vi "Set Temp Value.vi"(8 "error in (no error)":errorcluster, 10 "Temp.":dbl, 11 "Central Control in":refnum<class "Central Control.lvclass">) -> (0 "error out":errorcluster, 3 "Central Control out":refnum<class "Central Control.lvclass">)   [LabVIEW 2021, in "Central Control.lvlib" / "Central Control.lvclass"]
uses:
  Central Control.lvclass
  Central Control.lvclass/Central Control.ctl
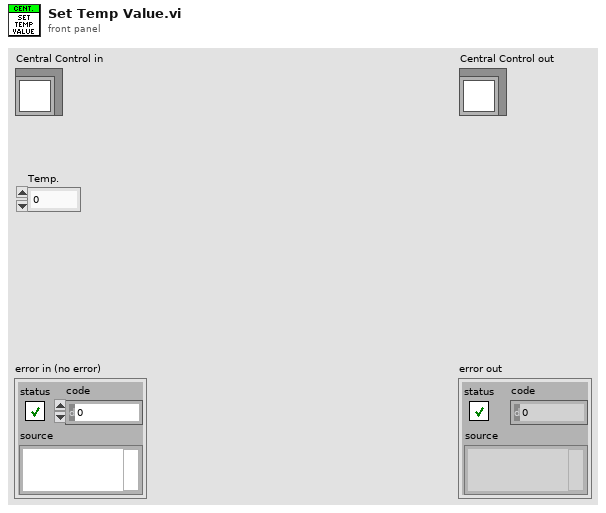
[diagram p1: front panel]
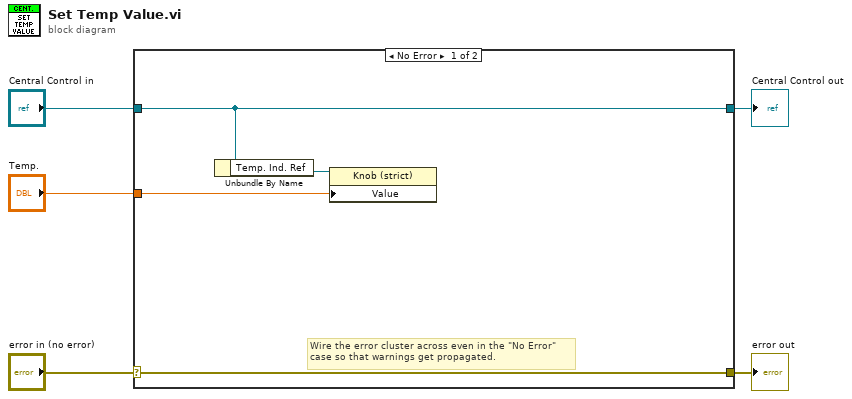
[diagram p0: block diagram]
diagram:
  n1 = case shown="No Error" "error in (no error)" {
    selector: "error in (no error)" -> [w9 w11]
    tunnel: [w9 w11] -> w4
    tunnel: [w8 w10] -> w2
    tunnel: "Central Control in" -> [w8 w10]
    tunnel: "Temp." -> [w6 _]
    frame No Error {
      # "Wire the error cluster across even in the \"No Error\"\ncase so that warnings get propagated."
      n2 = Unbundle By Name(w8) -> ("Temp. Ind. Ref"=w7:refnum<vi>)
      n3 = property class="Knob (strict)"(reference=w7, "Value"=w6) -> ()  [unwired: 1 in, 2 out]
    }
    frame Error {
    }
  }
  "error out" <- w4
  "Central Control out" <- w2
